vi "System Model.vi"() -> ()   [LabVIEW 2014]
uses:
  <vilib>/addons/Control Design/_Model Construction/Model Typedefs.llb/CD State Space Model (MIMO).ctl
  <vilib>/addons/Control Design/_Model Construction/Model Typedefs.llb/CD General Elements.ctl
  <vilib>/addons/Control Design/_Utility/Model Viewer.llb/Model Viewer SubVI/CD State-Space Rendering Options.ctl
  <vilib>/addons/Control Design/_Dynamic Analysis/Dynamic Analysis.llb/Dynamic Analysis subVI/cd_DC Gain (State-Space).vi
  <vilib>/addons/Control Design/_Utility/Model Viewer.llb/Model Viewer SubVI/cd_Draw State-Space Equation (SS).vi
  <vilib>/addons/Control Design/_Utility/NI_CD_Model Viewer.lvlib
  <vilib>/addons/Control Design/_Dynamic Analysis/NI_CD_Dynamic Analysis.lvlib
  <vilib>/addons/Control Design/_Model Construction/NI_LinSys_Model Typedefs.lvlib
panel:
  out "DC Gain":dbl
  out "Draw Area Size":cluster{"Width":u32, "Height":u32}
  out "Equation":picture
  in  "State-Space Model":T1 {"Transport Delay" format="%.2f"; "D" format="%#.2g"; "C" format="%#.2g"; "B" format="%#.2g"; "A" format="%#.2g"; "properties"."Sampling Time" format="%#.6p"; "properties"."Output Delays" format="%.4f"; "properties"."Input Delays" format="%.4f"}
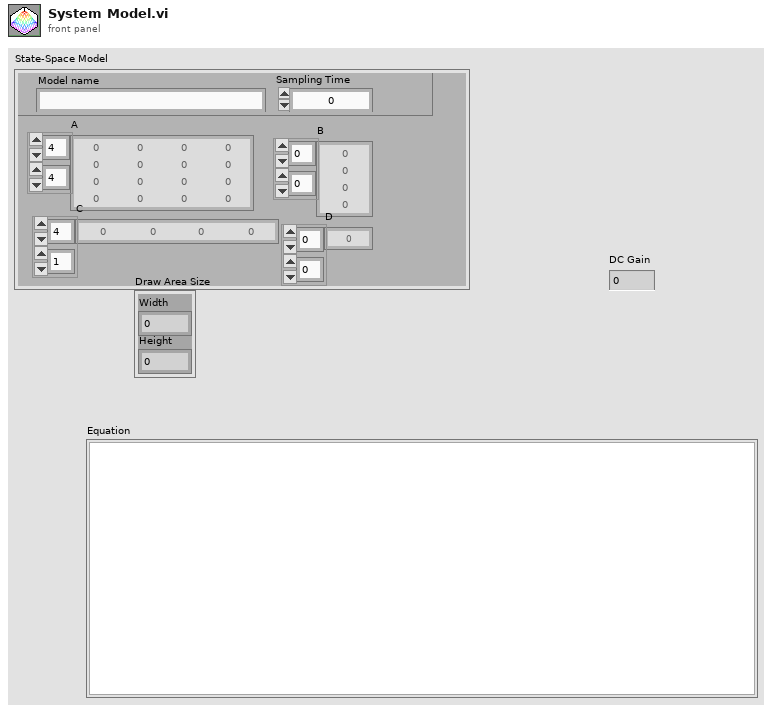
[diagram p1: front panel]
types:
  T1 = typedef "NI_LinSys_Model Typedefs.lvlib/CD State Space Model (MIMO).ctl" = cluster{"properties":T2, "A":dbl[][], "B":dbl[][], "C":dbl[][], "D":dbl[][], "StateNames":string[], "Transport Delay":dbl[][]}
  T2 = typedef "NI_LinSys_Model Typedefs.lvlib/CD General Elements.ctl" = cluster{"Model name":string, "Input names":string[], "Output names":string[], "Input Delays":dbl[], "Output Delays":dbl[], "Sampling Time":dbl, "Notes":string}
  T3 = typedef "NI_CD_Model Viewer.lvlib/CD State-Space Rendering Options.ctl" = u16
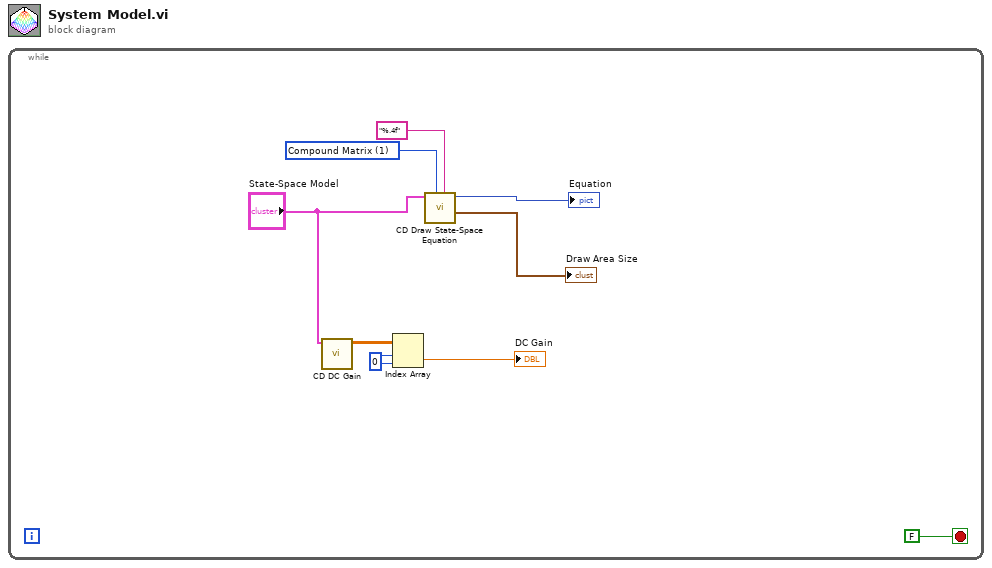
[diagram p0: block diagram]
diagram:
  n1 = while {
    stop <- FALSE stop-if-true
    w3 = 0 ("disabled index (col)")
    w9 = T3 1 items=["Equation", "Compound Matrix", "Quadruple"] ("Display Format")
    n2 = call-poly <vilib>:"CD DC Gain.vi"("State-Space Model"="State-Space Model") -> ("DC Gain"=w4:dbl[][])  [unwired: 8 in, 2 out]
    n3 = Index Array(array=w4, index (row)=w3, index (col)=w3) -> (element=→"DC Gain":dbl)
    n4 = call-poly <vilib>:"CD Draw State-Space Equation.vi"("Format Coefficients"="%.4f", "Display Format"=w9, "State-Space Model"="State-Space Model") -> ("Draw Area Size"=→"Draw Area Size":cluster{"Width":u32, "Height":u32}, "Equation"=→"Equation":picture)  [unwired: 6 in, 1 out]
  }
